vi "UpdateState2.vi"(0 "XRef":T9, 1 "Old State":T8, 2 "Version":T6) -> (14 "Is Good?":T5, 15 "Reply":T3, 16 "Fatal Error Out":T2, 17 "State Out":T1)   [LabVIEW 2014, in "RefManager(dev).lvlib" / "refmgr_get.xnode"]
uses:
  refmgr_get.xnode
  <vilib>/XNodeSupport/XNodeXNodeRef.ctl
  <vilib>/XNodeSupport/XNodeVariant.ctl
  <vilib>/XNodeSupport/XNodeVersion.ctl
  <vilib>/XNodeSupport/XNodeUShort.ctl
  <vilib>/XNodeSupport/XNodeBool.ctl
  <vilib>/XNodeSupport/XNodeStringArray.ctl
  <vilib>/XNodeSupport/XNodeString.ctl
  <vilib>/XNodeSupport/XNodeErrorCluster.ctl
  State.ctl
  <vilib>/XNodeSupport/NI_XNodeSupport.lvlib
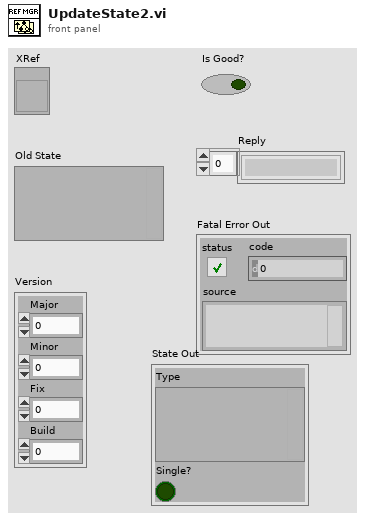
[diagram p1: front panel]
types:
  T1 = typedef "RefManager(dev).lvlib/refmgr_get.xnode/State.ctl" = cluster{"Type":variant, "Single?":bool}
  T2 = typedef "NI_XNodeSupport.lvlib/XNodeErrorCluster.ctl" = errorcluster
  T3 = typedef "NI_XNodeSupport.lvlib/XNodeStringArray.ctl" = T4[]
  T4 = typedef "NI_XNodeSupport.lvlib/XNodeString.ctl" = string
  T5 = typedef "NI_XNodeSupport.lvlib/XNodeBool.ctl" = bool
  T6 = typedef "NI_XNodeSupport.lvlib/XNodeVersion.ctl" = cluster{"Major":T7, "Minor":T7, "Fix":T7, "Build":T7}
  T7 = typedef "NI_XNodeSupport.lvlib/XNodeUShort.ctl" = u16
  T8 = typedef "NI_XNodeSupport.lvlib/XNodeVariant.ctl" = variant
  T9 = typedef "NI_XNodeSupport.lvlib/XNodeXNodeRef.ctl" = refnum<vi>
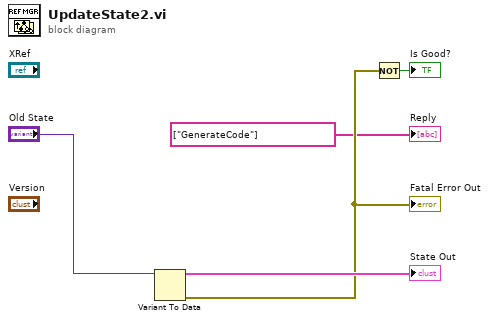
[diagram p0: block diagram]
diagram:
  n1 = Variant To Data(Variant="Old State") -> (data=→"State Out":T1, error out=w3:errorcluster)  [unwired: 2 in]
  "Fatal Error Out" <- w3
  n2 = Not(x=w3) -> (.not. x?=→"Is Good?":bool)
  "Reply" <- T3 ["GenerateCode"] ("Reply")
